vi "Test_Waves.vi"() -> ()   [LabVIEW 2015]
uses:
  <vilib>/addons/database/_DB Variant To Data/Database Variant To Data.xnode
panel:
  in  "Continue":bool
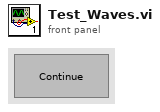
[diagram p1: front panel]
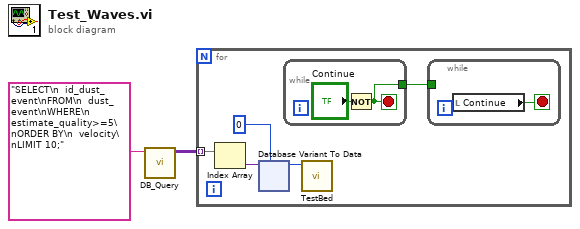
[diagram p0: block diagram]
diagram:
  n1 = call "DB_Query.vi"("Parameterized Query"="SELECT\n  id_dust_event\nFROM\n  dust_event\nWHERE\n  estimate_quality>=5\nORDER BY\n  velocity\nLIMIT 10;" ("format string")) -> ("Results"=w2:variant[][])  [unwired: 8 in, 2 out]
  n2 = for {
    tunnel: w2 -> [w7] mode=indexing
    n3 = Index Array(array=w7) -> (element=w6:variant)  [unwired: 1 in]
    n4 = xnode "Database Variant To Data"("database variant"=w6, "type"=0) -> ("data"=w4:i32)  [unwired: 1 in, 1 out]
    n5 = while {
      tunnel: [w9] -> w3
      stop <- w9 stop-if-true
      n6 = Not(x="Continue") -> (.not. x?=w9:bool)
    }
    n7 = call "TestBed.vi"("Dust ID"=w4) -> ()  [unwired: 11 in]
    n8 = while {
      tunnel: w3 -> [_]
      stop <- w8 stop-if-true
      n9 = local read "Continue"() -> (w8:bool)
    }
  }
